vi "PigeonIMU TESTER.vi"() -> ()   [LabVIEW 2023]
uses:
  Cluster_CMD_SEN_Data.ctl
  Shared Code/TypeDefs/Cluster_Unity Yaw-Pitch-Roll.ctl
  Shared Code/TypeDefs/Dial_Compase heading unit circle CCW positive.ctl
  RoboRIO Utilities/Global_STOP.vi
  Global_CMD_SEN_Data In.vi
  Global_SEN_Data Out.vi
  PigeonIMU_SEN_ts.lvlib
panel:
  out "Unit Yaw-Pitch-Roll":T1 {"Roll" scale format="%.3f"; "Pitch" scale format="%.3f"; "Yaw" scale format="%.3f"}
  in  "Update Rate (ms)":u32=100
  in  "Send Command":bool
  in  "CMD Cluster":T3
  in  "Finish":bool
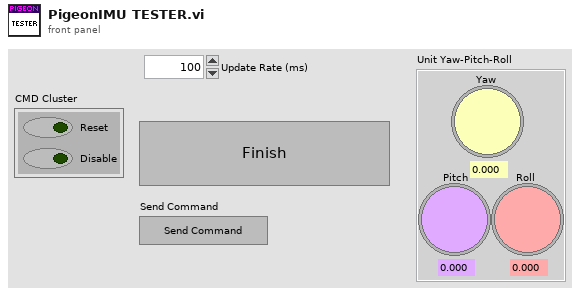
[diagram p1: front panel]
types:
  T1 = typedef "Cluster_Unity Yaw-Pitch-Roll.ctl" = cluster{"Yaw":T2, "Pitch":T2, "Roll":T2}
  T2 = typedef "Dial_Compase heading unit circle CCW positive.ctl" = dbl
  T3 = typedef "PigeonIMU_SEN_ts.lvlib/Cluster_CMD_SEN_Data.ctl" = cluster{"Reset":bool, "Disable":bool}
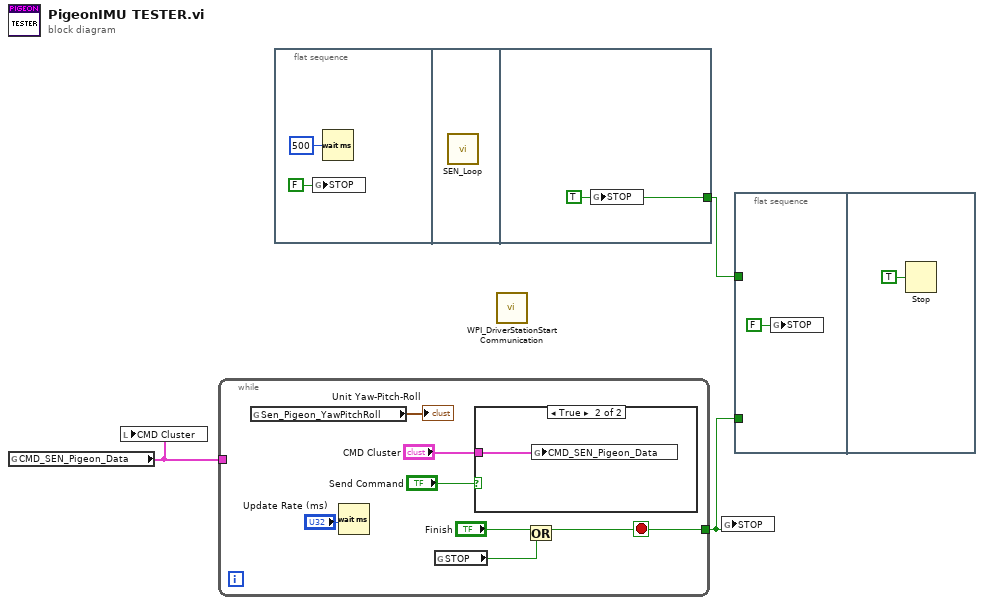
[diagram p0: block diagram]
diagram:
  n1 = global read "Global_CMD_SEN_Data In.vi" "CMD_SEN_Pigeon_Data"() -> (w1:T3)
  n2 = local write "CMD Cluster"(w1) -> ()
  n3 = while {
    tunnel: [w6] -> w3
    tunnel: w1 -> [_]
    stop <- w6 stop-if-true
    n4 = global read "Global_SEN_Data Out.vi" "Sen_Pigeon_YawPitchRoll"() -> (→"Unit Yaw-Pitch-Roll":T1)
    n5 = Wait (ms)(milliseconds to wait="Update Rate (ms)") -> ()  [unwired: 1 out]
    n6 = global read "Global_STOP.vi" "STOP"() -> (w5:bool)
    n7 = case shown="True" "Send Command" {
      tunnel: "CMD Cluster" -> [_ w11]
      frame False {
      }
      frame True {
        n8 = global write "Global_CMD_SEN_Data In.vi" "CMD_SEN_Pigeon_Data"(w11) -> ()
      }
    }
    n9 = Or(x="Finish", y=w5) -> (x .or. y?=w6:bool)
  }
  n10 = flat-sequence {
    tunnel: [w14] -> w2
    frame #0 {
      n11 = global write "Global_STOP.vi" "STOP"(FALSE ("STOP")) -> ()
      n12 = Wait (ms)(milliseconds to wait=u32 500) -> ()  [unwired: 1 out]
    }
    frame #1 {
      n13 = call "SEN_Loop.vi"() -> ()  [unwired: 12 in]
    }
    frame #2 {
      w14 = TRUE ("STOP")
      n14 = global write "Global_STOP.vi" "STOP"(w14) -> ()
    }
  }
  n15 = call <vilib>:"WPI_DriverStationStart Communication.vi"() -> ()  [unwired: 3 in, 9 out]
  n16 = global write "Global_STOP.vi" "STOP"(w3) -> ()
  n17 = flat-sequence {
    tunnel: w3 -> [_]
    tunnel: w2 -> [_]
    frame #0 {
      n18 = global write "Global_STOP.vi" "STOP"(FALSE ("STOP")) -> ()
    }
    frame #1 {
      n19 = Stop(stop? (T)=TRUE) -> ()
    }
  }
